vi "Construct.vi"(0 "iUser Configuration Manager in":refnum<class "iUser Configuration Manager.lvclass">, 5 "Encryption Type":refnum<class "iEncryption.lvclass">, 11 "error in":errorcluster) -> (4 "dup iUser Configuration Manager DVR":refnum<data-value>, 15 "error out":errorcluster)   [LabVIEW 2017, in "User Configuration Manager.lvlib" / "By Ref.lvlib"]
uses:
  <vilib>/gpm_packages/@cs/user-manager/Source/User Configuration Manager Ref/By Ref.lvlib
  <vilib>/gpm_packages/@cs/user-manager/Source/iUser Configuration Manager/iUser Configuration Manager.lvclass
  <vilib>/gpm_packages/@cs/user-manager/Source/iEncryption/iEncryption.lvclass
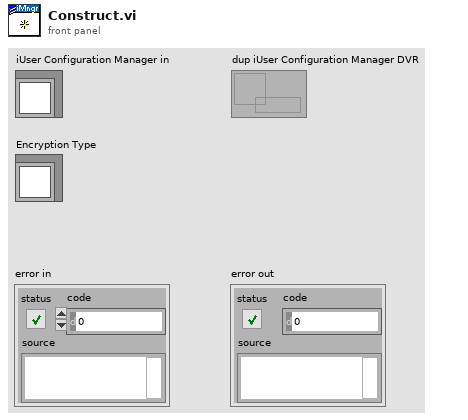
[diagram p1: front panel]
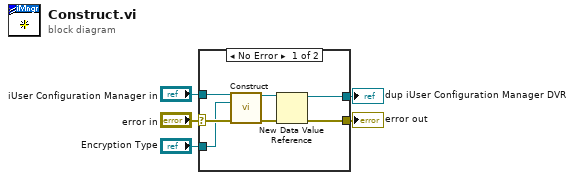
[diagram p0: block diagram]
diagram:
  n1 = case shown="No Error" "error in" {
    selector: "error in" -> [w12 w13]
    tunnel: [w9 w13] -> w5
    tunnel: [w11 _] -> w3
    tunnel: "iUser Configuration Manager in" -> [w8 _]
    tunnel: "Encryption Type" -> [w6 _]
    frame No Error {
      n2 = call-dynamic "Construct.vi"("iUser Configuration Manager in"=w8, "Encryption Type"=w6, "error in (no error)"=w12) -> ("iUser Configuration Manager out"=w7:refnum<class "iUser Configuration Manager.lvclass">, "error out"=w10:errorcluster)  [unwired: 11 in]
      n3 = New Data Value Reference(data value=w7, error in=w10) -> (data value reference=w11:refnum<data-value>, error out=w9:errorcluster)
    }
    frame Error {
    }
  }
  "error out" <- w5
  "dup iUser Configuration Manager DVR" <- w3
